vi "DefaultFromINI.vi"(8 "error in (no error)":errorcluster, 11 "ChromaPowerSupply":refnum<class "ChromaPowerSupply.lvclass">) -> (0 "error out":errorcluster, 3 "ChromaPowerSupply":refnum<class "ChromaPowerSupply.lvclass">)   [LabVIEW 2018, in "AcPwrPlugins.lvlib" / "ChromaPowerSupply.lvclass"]
doc: "This VI loads the instruments' configuration previously stored on file."
uses:
  ChromaPowerSupply.lvclass
  C:/Program Files (x86)/National Instruments/LabVIEW 2018/user.lib/NIST/BaseClasses/BasePlugin_class/BasePlugin.lvclass
  C:/Projects/ICDAS/NistPluggableModules/AcPwr/AcPwrPlugins/AcPwrBaseClass/AcPwrBase.lvclass
  TypeDefs/Device(s)Settings.ctl
  TypeDefs/Measurements.ctl
  <userlib>/NIST/BaseClasses/BasePlugin_class/BasePlugin.lvclass/BasePlugin.ctl
  <userlib>/NIST/BaseClasses/BasePlugin_class/Accessors/Read PluginIniFilePath.vi
  AcPwrBaseClass/AcPwrBase.lvclass
  <vilib>/Utility/config.llb/NI_LVConfig.lvlib
  TestClass/Test.lvclass
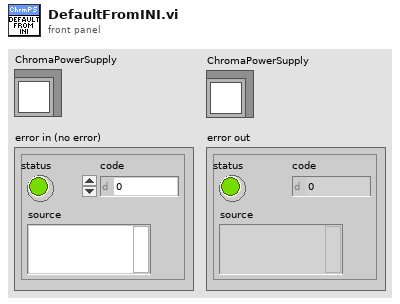
[diagram p1: front panel]
types:
  T1 = typedef "AcPwrPlugins.lvlib/ChromaPowerSupply.lvclass/Measurements.ctl" = cluster{"Handle":string, "Name":string, "Enabled":bool, "Measurement Value":dbl, "btnMeasFetch":bool, "ProtectionStatusString":string, "Measurement Type":enum16{"Voltage", "Current", "Power"}}[]
  T2 = typedef "AcPwrPlugins.lvlib/ChromaPowerSupply.lvclass/Device(s)Settings.ctl" = cluster{"Phases":cluster{"Handle":string, "Instrument Options":string, "id query (T)":bool, "reset device (T)":bool, "Timing":cluster{"TimingOn":enum16{""}, "Hours":u32, "Minutes":u32, "Seconds":dbl, "CutoffVoltage":dbl}, "Connected":bool, "Output Mode":enum16{"Voltage (DC)", "Current (DC)"}, "Voltage":dbl, "Current":dbl, "High Voltage Limit":dbl, "High Current Limit":dbl, "Power Protect":dbl, "Current Protect":dbl, "Voltage Protect":dbl, "Low Current Limit":dbl, "Low Voltage Limit":dbl, "Current Slew Rate":dbl, "Voltage Slew Rate":dbl, "Current Slew Infinite?":bool}[], "MeasName":string}
  T3 = typedef "NI_LVConfig.lvlib/Config Data RefNum.ctl" = refnum<k1>
  T4 = typedef "Test.lvclass/INIInfo.ctl" = cluster{"Module Name":string, "INI File Name":string, "Class Name":string, "INI File Name Without Extension":string, "Module.Class.INI File Name":string, "Visualization VI Path":path, "Instrument Class Path":path}
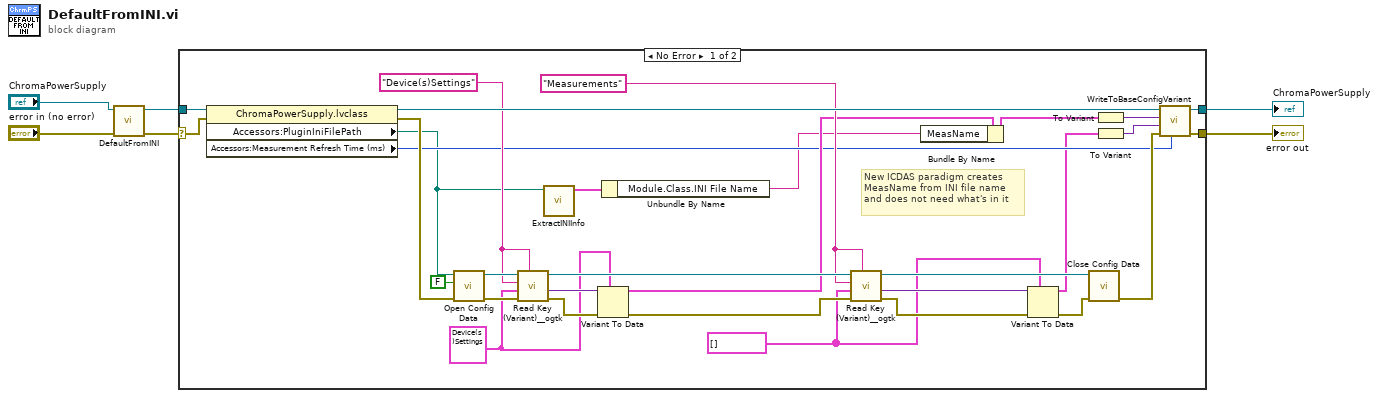
[diagram p0: block diagram]
diagram:
  n1 = call-parent "DefaultFromINI.vi"("error in (no error)"="error in (no error)", "AcPwrBase"="ChromaPowerSupply") -> ("error out"=w4:errorcluster, "AcPwrBase"=w3:refnum<class "ChromaPowerSupply.lvclass">)  [unwired: 8 in]
  n2 = case shown="No Error" w4 {
    selector: w4 -> [w29 w38]
    tunnel: w3 -> [w37 w39]
    tunnel: [w18 w39] -> w2
    tunnel: [w17 w38] -> w1
    frame No Error {
      w12 = T1 [] ("Measurements")
      w13 = T2 {"Phases"=[{"Handle"="", "Instrument Options"="", "id query (T)"=TRUE, "reset device (T)"=TRUE, "Timing"={"TimingOn"=enum."", "Hours"=0, "Minutes"=0, "Seconds"=0.0, "CutoffVoltage"=0.0}, "Connected"=FALSE, "Output Mode"=enum."Voltage (DC)", "Voltage"=0.0, "Current"=0.0, "High Voltage Limit"=0.0, "High Current Limit"=0.0, "Power Protect"=0.0, "Current Protect"=0.0, "Voltage Protect"=0.0, "Low Current Limit"=0.0, "Low Voltage Limit"=0.0, "Current Slew Rate"=0.0, "Voltage Slew Rate"=0.0, "Current Slew Infinite?"=TRUE}], "MeasName"=""} ("Device(s)Settings")
      w20 = "Measurements" ("section")
      w30 = "Device(s)Settings" ("section")
      # "New ICDAS paradigm creates\nMeasName from INI file name\nand does not need what's in it"
      n3 = property class="ChromaPowerSupply.lvclass"(reference=w37, error in=w29) -> (reference out=w31:refnum<class "ChromaPowerSupply.lvclass">, error out=w28:errorcluster, "Accessors:PluginIniFilePath"=w11:path, "Accessors:Measurement Refresh Time (ms)"=w15:u32)
      n4 = call <vilib>:"Open Config Data.vi"("error in (no error)"=w28, "create file if necessary (T)"=FALSE, "configuration file path"=w11) -> ("error out"=w34:errorcluster, "refnum"=w35:T3)  [unwired: 6 in, 1 out]
      n5 = call <userlib>:"Read Key (Variant)__ogtk.vi"("section"=w30, "error in (no error)"=w34, "type"=w13, "key (optional)"=w30, "refnum"=w35) -> ("error out"=w32:errorcluster, "key-value"=w33:variant, "refnum out"=w24:T3)  [unwired: 3 in, 1 out]
      n6 = call "ExtractINIInfo.vi"("INI File Path"=w11) -> ("INI Info"=w8:T4)  [unwired: 8 in, 2 out]
      n7 = Variant To Data(error in=w32, type=w13, Variant=w33) -> (data=w16:T2, error out=w21:errorcluster)
      n8 = Unbundle By Name(w8) -> ("Module.Class.INI File Name"=w7:string)
      n9 = call <userlib>:"Read Key (Variant)__ogtk.vi"("section"=w20, "error in (no error)"=w21, "type"=w12, "key (optional)"=w20, "refnum"=w24) -> ("error out"=w26:errorcluster, "key-value"=w25:variant, "refnum out"=w23:T3)  [unwired: 3 in, 1 out]
      n10 = Bundle By Name(cluster=w16, "MeasName"=w7) -> (w9:T2)
      n11 = Variant To Data(error in=w26, type=w12, Variant=w25) -> (data=w10:T1, error out=w22:errorcluster)
      n12 = call <vilib>:"Close Config Data.vi"("error in (no error)"=w22, "refnum"=w23) -> ("error out"=w27:errorcluster)  [unwired: 8 in, 1 out]
      n13 = To Variant(anything=w9) -> (Variant=w19:variant)
      n14 = To Variant(anything=w10) -> (Variant=w14:variant)
      n15 = call-dynamic "WriteToBaseConfigVariant.vi"("Measurement Refresh Time (ms)"=w15, "error in (no error)"=w27, "Meas"=w14, "Config"=w19, "ChromaPowerSupply in"=w31) -> ("error out"=w17:errorcluster, "ChromaPowerSupply out"=w18:refnum<class "ChromaPowerSupply.lvclass">)  [unwired: 5 in]
    }
    frame Error {
    }
  }
  "error out" <- w1
  "ChromaPowerSupply" <- w2
